vi "EditUser.vi"(11 "error in (no error)":errorcluster) -> (15 "error out":errorcluster)   [LabVIEW 2021]
panel:
  in  "Cancel":bool
  in  "New Password":string
  in  "Select User":string(combo)
  in  "UpdatePassword":bool
  in  "Help":bool
  # "Edit Password"
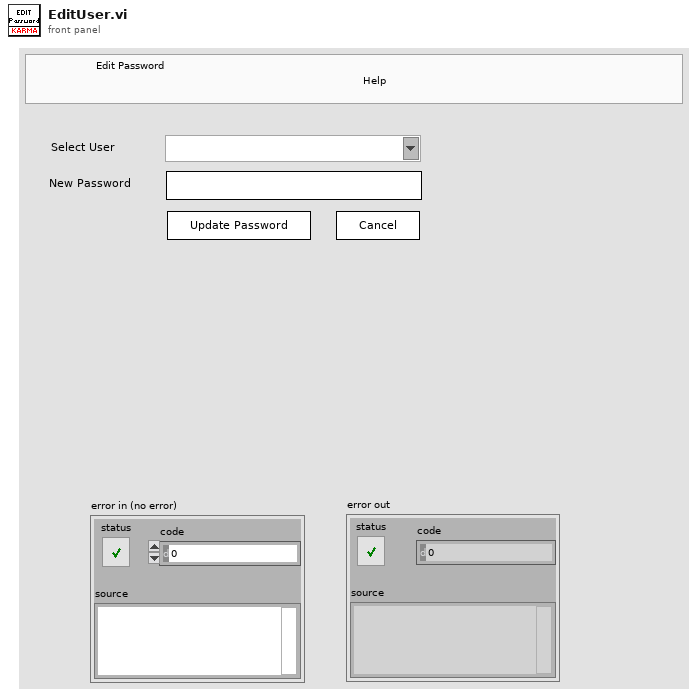
[diagram p1: front panel]
types:
  T1 = enum16{"Poll", "Initialize", "UpdatePassword", "Error", "Exit"}
  T2 = typedef "UserInfo.ctl" = cluster{"User Name":string, "Password":string, "UserType":T3}
  T3 = typedef "UserTypes.ctl" = u16
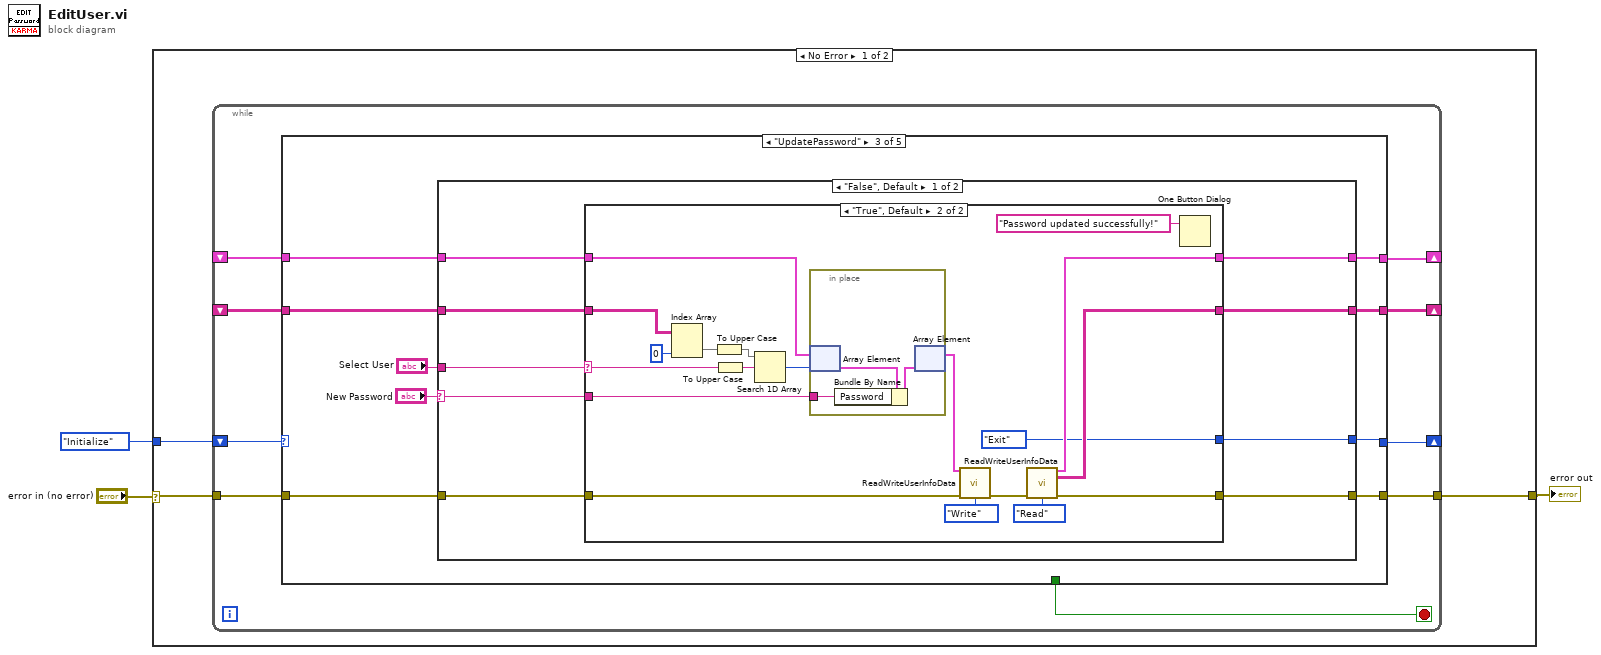
[diagram p0: block diagram]
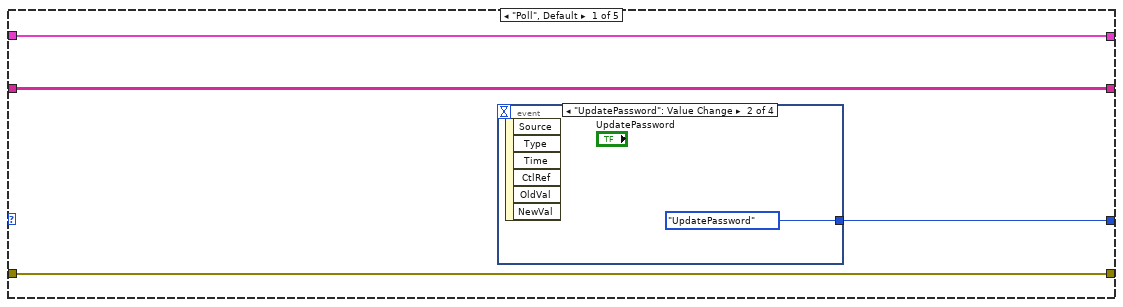
[diagram p2: hidden frame]
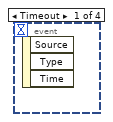
[diagram p3: hidden frame]
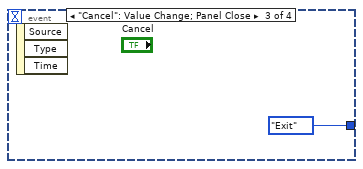
[diagram p4: hidden frame]
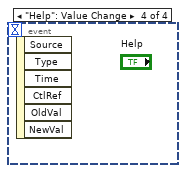
[diagram p5: hidden frame]
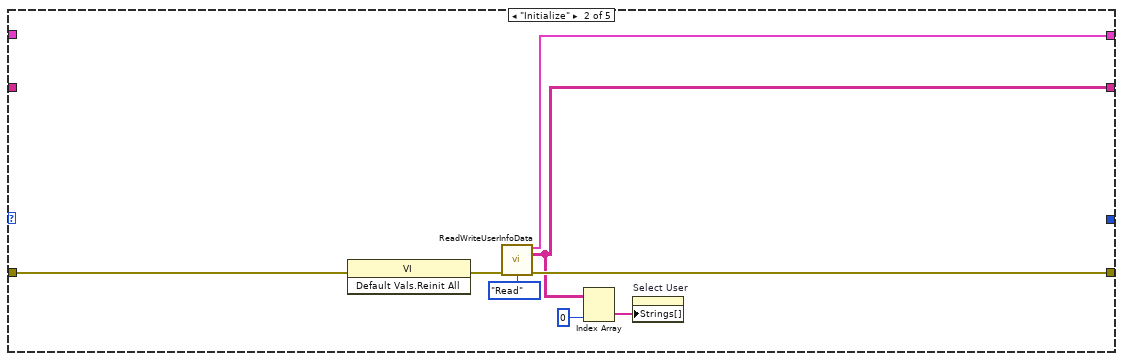
[diagram p6: hidden frame]
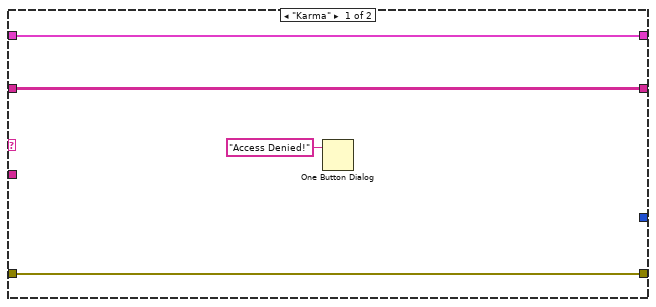
[diagram p7: hidden frame]
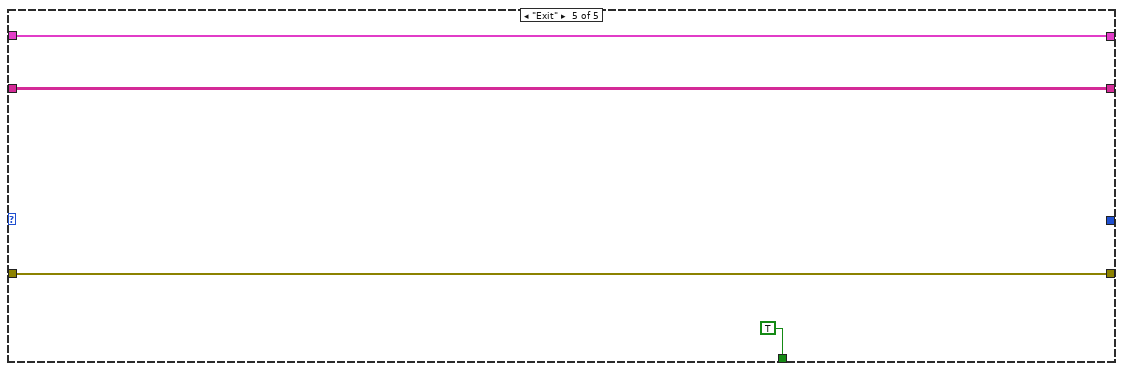
[diagram p10: hidden frame]
diagram:
  n1 = case shown="No Error" "error in (no error)" {
    selector: "error in (no error)" -> [w6 w84]
    tunnel: [w5 w84] -> w2
    tunnel: T1."Initialize" -> [w4 _]
    frame No Error {
      n2 = while {
        tunnel: w6 -> [w15]
        tunnel: [w14] -> w5
        shift-right: [w12] -> _
        shift-left: w4 -> [w13]
        shift-right: [w10] -> _
        shift-left: _ -> [w8]
        shift-right: [w9] -> _
        shift-left: _ -> [w7]
        stop <- w11 stop-if-true
        n3 = case shown="\"UpdatePassword\"" w13 {
          tunnel: w15 -> [w19 w26 w34 w79 w83]
          tunnel: [w19 w25 w33 w79 w83] -> w14
          tunnel: [w18 _ w30 _ _] -> w12
          tunnel: [_ _ _ _ TRUE] -> w11
          tunnel: [w16 w23 w32 w77 w80] -> w10
          tunnel: [w17 w22 w31 w78 w81] -> w9
          tunnel: w8 -> [w16 _ w38 w77 w80]
          tunnel: w7 -> [w17 _ w35 w78 w81]
          frame "Poll", Default {
            n4 = event shown="[1] \"UpdatePassword\": Value Change" {
              selector: _ -> [_ _ _ _]
              dyn-events: _ -> [_ _ _ _]
              timeout: _ -> [_ _ _ _]
              tunnel: [_ T1."UpdatePassword" T1."Exit" _] -> w18
              event Timeout {
                n5 = event-data() -> ()  [unwired: 1 in, 3 out]
              }
              event "UpdatePassword": Value Change {
                n6 = event-data() -> ()  [unwired: 1 in, 6 out]
              }
              event "Cancel": Value Change; Panel Close {
                n7 = event-data() -> ()  [unwired: 1 in, 3 out]
              }
              event "Help": Value Change {
                n8 = event-data() -> ()  [unwired: 1 in, 6 out]
              }
            }
          }
          frame "Initialize" {
            n9 = invoke class="VI" method="Default Vals.Reinit All"(error in=w26) -> (error out=w27:errorcluster)  [unwired: 2 in, 2 out]
            n10 = call "ReadWriteUserInfoData.vi"("Error in (no error)"=w27, "Operation"=enum16{"Write", "Read"}."Read") -> ("User Info Array of Clusters Out"=w22:T2[], "User Info Array out"=w23:string[][], "Error out"=w25:errorcluster)  [unwired: 11 in]
            n11 = Index Array(array=w23, index (col)=0 ("disabled index (col)")) -> (element=w24:string[])  [unwired: 1 in]
            n12 = property on="Select User" class="CmbBox"("Strings[]"=w24) -> ()  [unwired: 2 in, 2 out]
          }
          frame "UpdatePassword" {
            n13 = case shown="\"False\", Default" "New Password" {
              selector: "New Password" -> [w45 _]
              tunnel: w38 -> [w47 w75]
              tunnel: "Select User" -> [w39 _]
              tunnel: w35 -> [w46 w76]
              tunnel: w34 -> [w44 w74]
              tunnel: [w43 w74] -> w33
              tunnel: [w42 w75] -> w32
              tunnel: [w41 w76] -> w31
              tunnel: [w40 _] -> w30
              frame "False", Default {
                n14 = case shown="\"True\", Default" w39 {
                  selector: w39 -> [_ w52]
                  tunnel: w47 -> [w50 w70]
                  tunnel: w46 -> [w51 w65]
                  tunnel: w45 -> [_ w63]
                  tunnel: w44 -> [w48 w58]
                  tunnel: [w48 w57] -> w43
                  tunnel: [w50 w55] -> w42
                  tunnel: [w51 w54] -> w41
                  tunnel: [_ T1."Exit"] -> w40
                  frame "Karma" {
                    n15 = One Button Dialog(message="Access Denied!") -> ()  [unwired: 1 in, 1 out]
                  }
                  frame "True", Default {
                    n16 = Index Array(array=w70, index (col)=0 ("disabled index (col)")) -> (element=w68:string[])  [unwired: 1 in]
                    n17 = To Upper Case(1:w68) -> (0:w66:string[])
                    n18 = To Upper Case(1:w52) -> (0:w67:string)
                    n19 = Search 1D Array(1D array=w66, element=w67) -> (index of element=w64:i32)  [unwired: 1 in]
                    n20 = in-place {
                      in-place-border: w63 -> [w71]
                      n21 = in-place-array #1(w65, w64) -> (w73:T2)
                      n22 = Bundle By Name(cluster=w73, "Password"=w71) -> (w72:T2)
                      n23 = in-place-array #1(w72) -> (w60:T2[])  [unwired: 1 out]
                    }
                    n24 = call "ReadWriteUserInfoData.vi"("User Info  Array In"=w60, "Error in (no error)"=w58, "Operation"=enum16{"Write", "Read"}."Write") -> ("Error out"=w61:errorcluster)  [unwired: 10 in, 2 out]
                    n25 = call "ReadWriteUserInfoData.vi"("Error in (no error)"=w61, "Operation"=enum16{"Write", "Read"}."Read") -> ("User Info Array of Clusters Out"=w54:T2[], "User Info Array out"=w55:string[][], "Error out"=w57:errorcluster)  [unwired: 11 in]
                    n26 = One Button Dialog(message="Password updated successfully!") -> ()  [unwired: 1 in, 1 out]
                  }
                }
              }
              frame "" {
              }
            }
          }
          frame "Error" {
          }
          frame "Exit" {
          }
        }
      }
    }
    frame Error {
    }
  }
  "error out" <- w2
